vi "setuphardware.vi"(8 "error in (no error)":errorcluster, 10 "Camera Name":T1="S1019101", 11 "Imaging in":refnum<class "Imaging.lvclass">) -> (0 "error out":errorcluster, 3 "Imaging out":refnum<class "Imaging.lvclass">)   [LabVIEW 2014, in "Imaging.lvclass"]
uses:
  Imaging.lvclass
  <vilib>/userdefined/High Color/IMAQdx.ctl
  Imaging.lvclass/Imaging.ctl
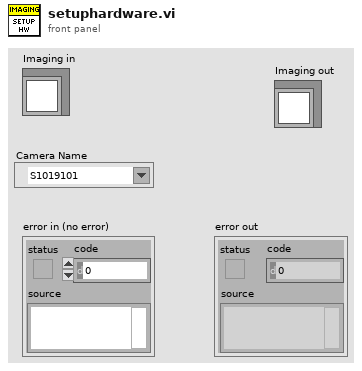
[diagram p1: front panel]
types:
  T1 = typedef "IMAQdx.ctl" = refnum<k21>
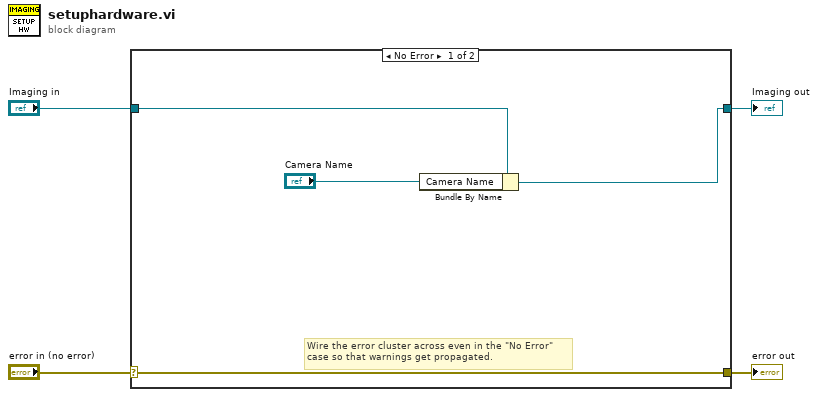
[diagram p0: block diagram]
diagram:
  n1 = case shown="No Error" "error in (no error)" {
    selector: "error in (no error)" -> [w8 w10]
    tunnel: [w8 w10] -> w3
    tunnel: [w6 w9] -> w1
    tunnel: "Imaging in" -> [w7 w9]
    frame No Error {
      # "Wire the error cluster across even in the \"No Error\"\ncase so that warnings get propagated."
      n2 = Bundle By Name(cluster=w7, "Camera Name"="Camera Name") -> (w6:refnum<class "Imaging.lvclass">)
    }
    frame Error {
    }
  }
  "error out" <- w3
  "Imaging out" <- w1
